vi "mainVI_MODCA.vi"() -> ()   [LabVIEW 2019]
panel:
  out "Graph":dbl[][](graph)
  in  "New plot":bool
  in  "stop":bool
  # "Make sure subVI front panel is clised before running this VI!"
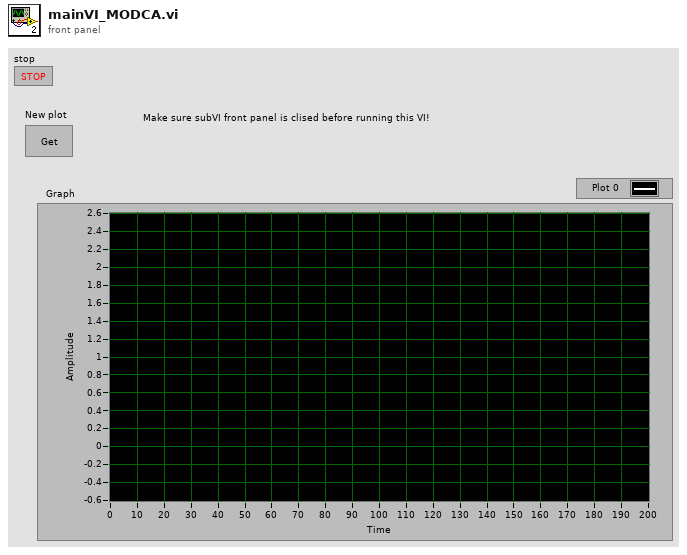
[diagram p1: front panel]
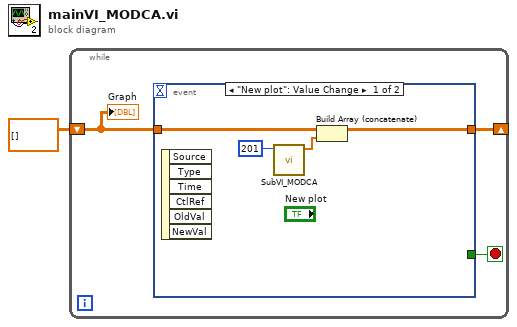
[diagram p0: block diagram]
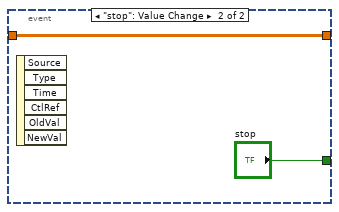
[diagram p2: hidden frame]
diagram:
  n1 = while {
    shift-right: [w4] -> _
    shift-left: dbl[][] [] -> [w3]
    stop <- w2 stop-if-true
    n2 = event shown="[0] \"New plot\": Value Change" {
      selector: _ -> [_ _]
      dyn-events: _ -> [_ _]
      timeout: _ -> [_ _]
      tunnel: [w6 w9] -> w4
      tunnel: w3 -> [w5 w9]
      tunnel: [_ "stop"] -> w2
      event "New plot": Value Change {
        n3 = event-data() -> ()  [unwired: 1 in, 6 out]
        n4 = call "SubVI_MODCA.vi"("Points"=201) -> ("Disorder Pattern"=w7:dbl[])  [unwired: 10 in]
        n5 = Build Array (concatenate)(w5, w7) -> (w6:dbl[][])
      }
      event "stop": Value Change {
        n6 = event-data() -> ()  [unwired: 1 in, 6 out]
      }
    }
    "Graph" <- w3
  }
